vi "CommentSequenceFile.vi"(10 "Configuration File Path":path=path "CommentSequenceFile.Sample.ini", 11 "Sequence Context":refnum<k7>) -> ()   [LabVIEW 2017]
uses:
  <vilib>/Utility/config.llb/Read Key (String).vi
  <vilib>/Utility/config.llb/NI_LVConfig.lvlib
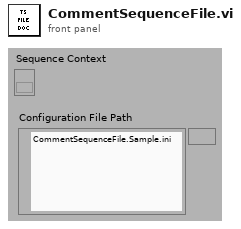
[diagram p1: front panel]
types:
  T1 = typedef "NI_LVConfig.lvlib/Config Data RefNum.ctl" = refnum<k1>
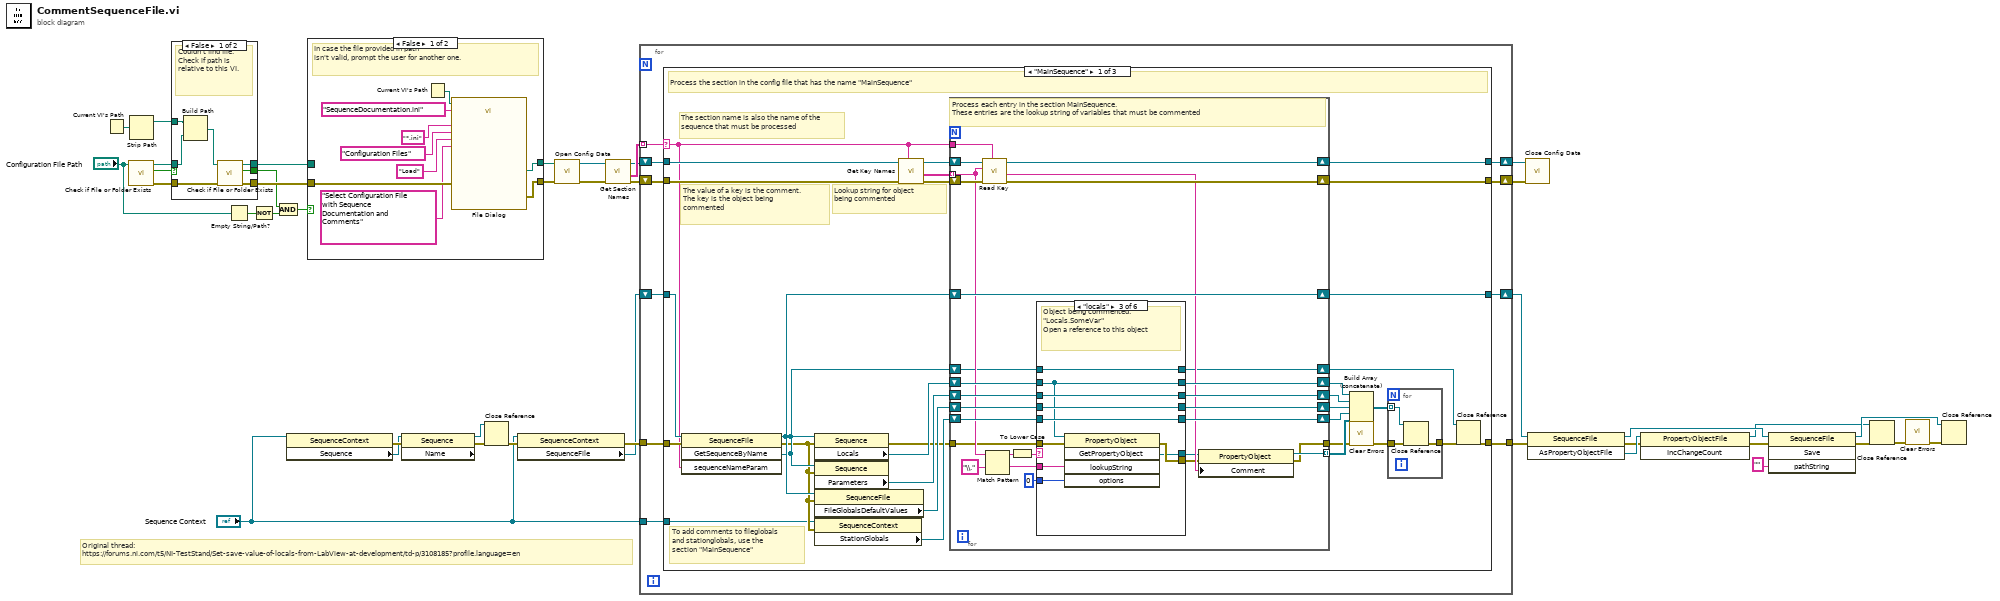
[diagram p0: block diagram]
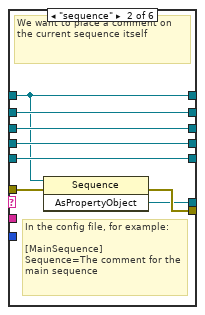
[diagram p4: hidden frame]
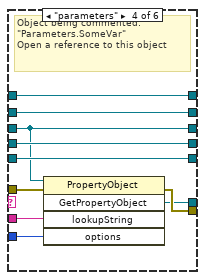
[diagram p5: hidden frame]
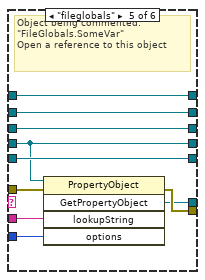
[diagram p6: hidden frame]
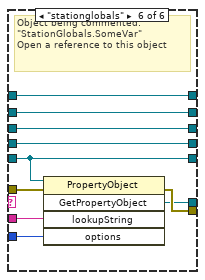
[diagram p7: hidden frame]
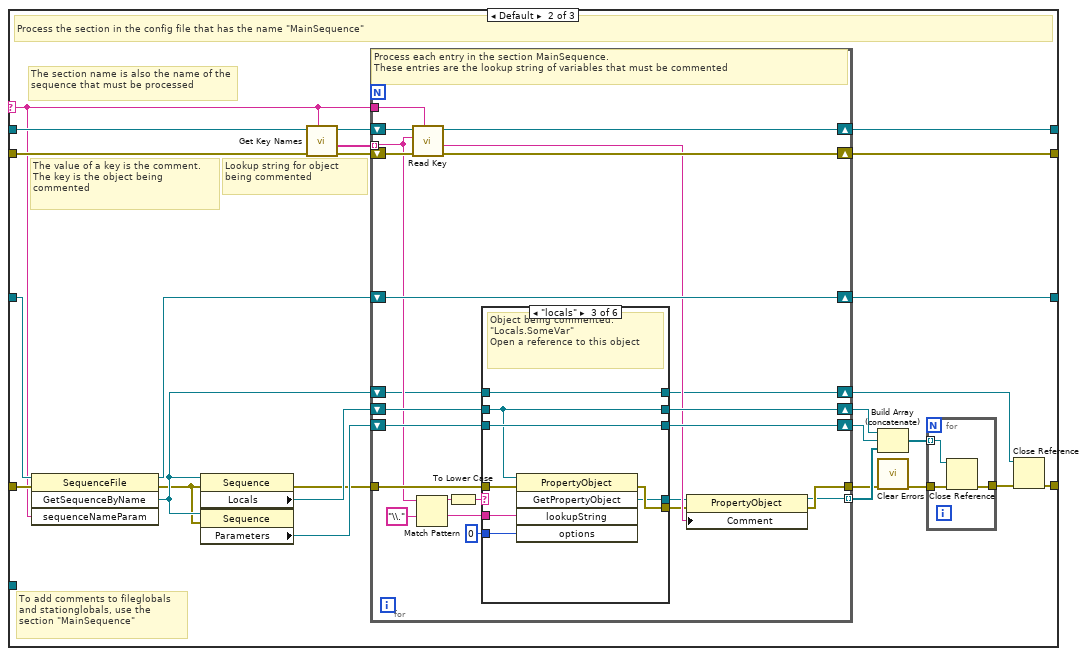
[diagram p8: hidden frame]
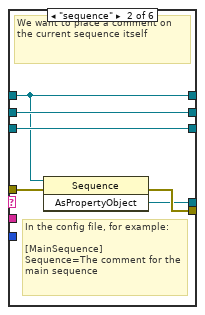
[diagram p10: hidden frame]
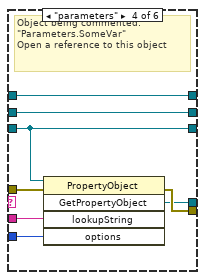
[diagram p11: hidden frame]
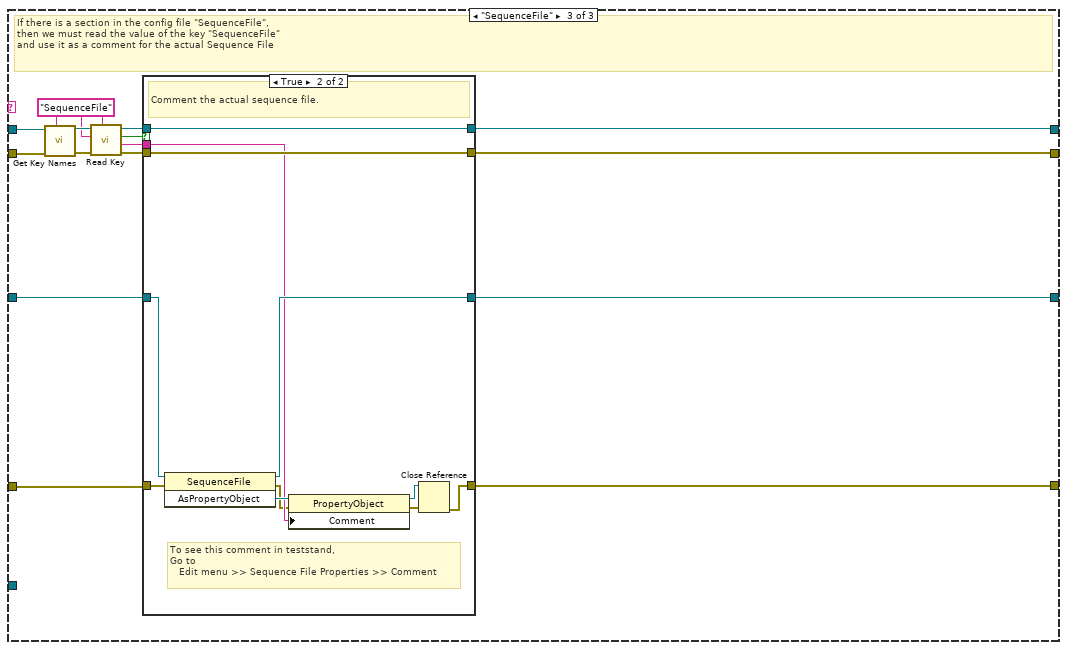
[diagram p14: hidden frame]
diagram:
  # "Original thread:\nhttps://forums.ni.com/t5/NI-TestStand/Set-save-value-of-locals-from-LabView-at-development/td-p/3108185?profile.language=en"
  n1 = Current VI's Path() -> (path=w2:path)
  n2 = call <vilib>:"Check if File or Folder Exists.vi"("path"="Configuration File Path") -> ("error out"=w7:errorcluster, "file or folder exists?"=w4:bool, "dup path"=w5:path)  [unwired: 8 in]
  n3 = Strip Path(path=w2) -> (stripped path=w1:path)  [unwired: 1 out]
  n4 = case shown="False" w4 {
    selector: w4 -> [_ w49]
    tunnel: [w46 w51] -> w8
    tunnel: w7 -> [w48 w51]
    tunnel: [w47 w50] -> w6
    tunnel: w5 -> [w43 w50]
    tunnel: [w45 w49] -> w3
    tunnel: w1 -> [w42 _]
    frame False {
      # "Couldn't find file.\nCheck if path is relative to this VI."
      n5 = Build Path(base path=w42, name or relative path=w43) -> (appended path=w44:path)
      n6 = call <vilib>:"Check if File or Folder Exists.vi"("error in (no error)"=w48, "path"=w44) -> ("error out"=w46:errorcluster, "file or folder exists?"=w45:bool, "dup path"=w47:path)  [unwired: 7 in]
    }
    frame True {
      # "Found file,\nNo worries"
    }
  }
  n7 = Empty String/Path?(string/path="Configuration File Path") -> (empty?=w12:bool)
  n8 = Not(x=w12) -> (.not. x?=w11:bool)
  n9 = And(x=w3, y=w11) -> (x .and. y?=w14:bool)
  n10 = property class="SequenceContext"(reference="Sequence Context") -> (error out=w30:errorcluster, "Sequence"=w24:refnum<k7>)  [unwired: 1 in, 1 out]
  n11 = case shown="False" w14 {
    tunnel: w6 -> [_ w62]
    tunnel: [w60 w62] -> w41
    tunnel: w8 -> [w58 w61]
    tunnel: [w59 w61] -> w40
    frame False {
      # "In case the file provided in path\nisn't valid, prompt the user for another one."
      n12 = Current VI's Path() -> (path=w57:path)
      n13 = call "File Dialog"("start path"=w57, "prompt"="Select Configuration File with Sequence Documentation and Comments", "button label"="Load", "default name"="SequenceDocumentation.ini", "error in"=w58, "pattern (all files)"="*.ini", "pattern label"="Configuration Files") -> ("selected path"=w60:path, "error out"=w59:errorcluster)  [unwired: 5 in, 2 out]
    }
    frame True {
      # "We have a valid file. No worries"
    }
  }
  n14 = property class="Sequence" props=["Name"](reference=w24, error in=w30) -> (reference out=w29:refnum<k7>, error out=w28:errorcluster)  [unwired: 1 out]
  n15 = Close Reference(reference=w29, error in (no error)=w28) -> (error out=w27:errorcluster)
  n16 = property class="SequenceContext"(reference="Sequence Context", error in=w27) -> (error out=w16:errorcluster, "SequenceFile"=w15:refnum<k7>)  [unwired: 1 out]
  n17 = call <vilib>:"Open Config Data.vi"("error in (no error)"=w40, "configuration file path"=w41) -> ("error out"=w21:errorcluster, "refnum"=w20:T1)  [unwired: 7 in, 1 out]
  n18 = call <vilib>:"Get Section Names.vi"("error in (no error)"=w21, "refnum"=w20) -> ("error out"=w17:errorcluster, "section names"=w19:string[], "refnum out"=w18:T1)  [unwired: 7 in]
  n19 = for {
    tunnel: "Sequence Context" -> [w68]
    shift-right: [w70] -> w25
    shift-left: w15 -> [w67]
    shift-right: [w72] -> w39
    shift-left: w17 -> [w65]
    shift-right: [w71] -> w38
    shift-left: w18 -> [w64]
    tunnel: w19 -> [w63] mode=indexing
    tunnel: w16 -> [w66]
    tunnel: [w69] -> w23
    n20 = case shown="\"MainSequence\"" w63 {
      selector: w63 -> [w79 w196 _]
      tunnel: [w102 w213 w278] -> w72
      tunnel: [w101 w212 w279] -> w71
      tunnel: [w98 w209 w277] -> w70
      tunnel: [w77 w193 w276] -> w69
      tunnel: w68 -> [w84 _ _]
      tunnel: w67 -> [w83 w200 w281]
      tunnel: w66 -> [w82 w199 w280]
      tunnel: w65 -> [w81 w198 w282]
      tunnel: w64 -> [w80 w197 w283]
      frame "MainSequence" {
        # "To add comments to fileglobals and stationglobals, use the section \"MainSequence\""
        # "Lookup string for object being commented"
        # "The value of a key is the comment. \nThe key is the object being commented"
        # "The section name is also the name of the sequence that must be processed"
        # "Process the section in the config file that has the name \"MainSequence\""
        n21 = invoke class="SequenceFile" method="GetSequenceByName"(reference=w83, error in=w82, "sequenceNameParam"=w79) -> (reference out=w96:refnum<k7>, error out=w85:errorcluster, "GetSequenceByName"=w86:refnum<k7>)  [unwired: 1 in, 1 out]
        n22 = property class="Sequence"(reference=w86, error in=w85) -> (error out=w75:errorcluster, "Locals"=w97:refnum<k7>)  [unwired: 1 out]
        n23 = property class="Sequence"(reference=w86, error in=w85) -> ("Parameters"=w95:refnum<k7>)  [unwired: 2 out]
        n24 = property class="SequenceFile"(reference=w96, error in=w85) -> ("FileGlobalsDefaultValues"=w94:refnum<k7>)  [unwired: 2 out]
        n25 = property class="SequenceContext"(reference=w84, error in=w85) -> ("StationGlobals"=w93:refnum<k7>)  [unwired: 2 out]
        n26 = call <vilib>:"Get Key Names.vi"("section"=w79, "error in (no error)"=w81, "refnum"=w80) -> ("error out"=w103:errorcluster, "key names"=w99:string[], "refnum out"=w100:T1)  [unwired: 5 in, 1 out]
        n27 = for {
          shift-right: [w131] -> w102
          shift-left: w103 -> [w134]
          shift-right: [w132] -> w101
          shift-left: w100 -> [w133]
          tunnel: w99 -> [w116] mode=indexing
          tunnel: w79 -> [w130]
          shift-right: [w127] -> w98
          shift-left: w96 -> [w127]
          shift-right: [w126] -> w92
          shift-left: w97 -> [w125]
          shift-right: [w120] -> w91
          shift-left: w93 -> [w119]
          shift-right: [w121] -> w90
          shift-left: w94 -> [w122]
          shift-right: [w124] -> w89
          shift-left: w95 -> [w123]
          tunnel: [w115] -> w88 mode=indexing
          shift-right: [w110] -> w76
          shift-left: w86 -> [w109]
          tunnel: w75 -> [w108]
          tunnel: [w107] -> w73
          # "Process each entry in the section MainSequence. \nThese entries are the lookup string of variables that must be commented"
          n28 = call-poly <vilib>:"Read Key.vi"("section"=w130, "error in (no error)"=w134, "key"=w116, "refnum"=w133) -> ("error out"=w131:errorcluster, "value"=w117:string, "refnum out"=w132:T1)  [unwired: 4 in, 1 out]
          n29 = Match Pattern(string=w116, regular expression="\\.") -> (before substring=w128:string, after substring=w114:string)  [unwired: 1 in, 2 out]
          n30 = To Lower Case(string=w128) -> (all lower case string=w118:string)
          n31 = case shown="\"locals\"" w118 {
            tunnel: [w136 w147 w150 w167 w177 w188] -> w126
            tunnel: w125 -> [w136 w147 w150 w167 w177 w188]
            tunnel: [w140 w146 w157 w165 w176 w186] -> w124
            tunnel: w123 -> [w140 w146 w157 w165 w176 w186]
            tunnel: w122 -> [w139 w142 w151 w166 w170 w187]
            tunnel: [w139 w142 w151 w166 w170 w187] -> w121
            tunnel: [w138 w148 w158 w168 w178 w180] -> w120
            tunnel: w119 -> [w138 w148 w158 w168 w178 w180]
            tunnel: [w137 w144 w155 w163 w174 w184] -> w111
            tunnel: w108 -> [w137 w145 w156 w164 w175 w185]
            tunnel: w114 -> [_ _ w154 w162 w173 w183]
            tunnel: 0 ("options") -> [_ _ w153 w161 w172 w182]
            tunnel: [_ w143 w152 w160 w171 w181] -> w112
            tunnel: [w135 w141 w149 w159 w169 w179] -> w110
            tunnel: w109 -> [w135 w141 w149 w159 w169 w179]
            frame Default {
              # "The object being commented does not belong to locals, fileglobals, stationglobals, or parameters.\n\nNote that form of the lookup string (from the keys in config file) must be of the form e.g.\n\nLocals.SomeVariable"
            }
            frame "sequence" {
              # "In the config file, for example:\n\n[MainSequence]\nSequence=The comment for the main sequence"
              # "We want to place a comment on the current sequence itself"
              n32 = invoke class="Sequence" method="AsPropertyObject"(reference=w141, error in=w145) -> (error out=w144:errorcluster, "AsPropertyObject"=w143:refnum<k7>)  [unwired: 1 in, 1 out]
            }
            frame "locals" {
              # "Object being commented:\n\"Locals.SomeVar\"\nOpen a reference to this object"
              n33 = invoke class="PropertyObject" method="GetPropertyObject"(reference=w150, error in=w156, "lookupString"=w154, "options"=w153) -> (error out=w155:errorcluster, "GetPropertyObject"=w152:refnum<k7>)  [unwired: 1 in, 3 out]
            }
            frame "parameters" {
              # "Object being commented:\n\"Parameters.SomeVar\"\nOpen a reference to this object"
              n34 = invoke class="PropertyObject" method="GetPropertyObject"(reference=w165, error in=w164, "lookupString"=w162, "options"=w161) -> (error out=w163:errorcluster, "GetPropertyObject"=w160:refnum<k7>)  [unwired: 1 in, 3 out]
            }
            frame "fileglobals" {
              # "Object being commented:\n\"FileGlobals.SomeVar\"\nOpen a reference to this object"
              n35 = invoke class="PropertyObject" method="GetPropertyObject"(reference=w170, error in=w175, "lookupString"=w173, "options"=w172) -> (error out=w174:errorcluster, "GetPropertyObject"=w171:refnum<k7>)  [unwired: 1 in, 3 out]
            }
            frame "stationglobals" {
              # "Object being commented:\n\"StationGlobals.SomeVar\"\nOpen a reference to this object"
              n36 = invoke class="PropertyObject" method="GetPropertyObject"(reference=w180, error in=w185, "lookupString"=w183, "options"=w182) -> (error out=w184:errorcluster, "GetPropertyObject"=w181:refnum<k7>)  [unwired: 1 in, 3 out]
            }
          }
          n37 = property class="PropertyObject"(reference=w112, error in=w111, "Comment"=w117) -> (reference out=w115:refnum<k7>, error out=w107:errorcluster)
        }
        n38 = Build Array (concatenate)(w92, w89, w90, w91, w88) -> (w87:refnum<k7>[])
        n39 = call <vilib>:"Clear Errors.vi"("error in (no error)"=w73) -> ("error out"=w74:errorcluster)  [unwired: 5 in, 1 out]
        n40 = for {
          tunnel: w87 -> [w106] mode=indexing
          tunnel: w74 -> [w105]
          tunnel: [w104] -> w78
          n41 = Close Reference(reference=w106, error in (no error)=w105) -> (error out=w104:errorcluster)
        }
        n42 = Close Reference(reference=w76, error in (no error)=w78) -> (error out=w77:errorcluster)
      }
      frame Default {
        # "To add comments to fileglobals and stationglobals, use the section \"MainSequence\""
        # "Lookup string for object being commented"
        # "The value of a key is the comment. \nThe key is the object being commented"
        # "The section name is also the name of the sequence that must be processed"
        # "Process the section in the config file that has the name \"MainSequence\""
        n43 = invoke class="SequenceFile" method="GetSequenceByName"(reference=w200, error in=w199, "sequenceNameParam"=w196) -> (reference out=w207:refnum<k7>, error out=w201:errorcluster, "GetSequenceByName"=w202:refnum<k7>)  [unwired: 1 in, 1 out]
        n44 = property class="Sequence"(reference=w202, error in=w201) -> (error out=w195:errorcluster, "Locals"=w208:refnum<k7>)  [unwired: 1 out]
        n45 = property class="Sequence"(reference=w202, error in=w201) -> ("Parameters"=w206:refnum<k7>)  [unwired: 2 out]
        n46 = call <vilib>:"Get Key Names.vi"("section"=w196, "error in (no error)"=w198, "refnum"=w197) -> ("error out"=w214:errorcluster, "key names"=w210:string[], "refnum out"=w211:T1)  [unwired: 5 in, 1 out]
        n47 = for {
          shift-right: [w238] -> w213
          shift-left: w214 -> [w241]
          shift-right: [w239] -> w212
          shift-left: w211 -> [w240]
          tunnel: w210 -> [w226] mode=indexing
          tunnel: w196 -> [w237]
          shift-right: [w234] -> w209
          shift-left: w207 -> [w234]
          shift-right: [w233] -> w205
          shift-left: w208 -> [w232]
          shift-right: [w231] -> w204
          shift-left: w206 -> [w230]
          tunnel: [w224] -> w191 mode=indexing
          shift-right: [w219] -> w192
          shift-left: w202 -> [w218]
          tunnel: w195 -> [w228]
          tunnel: [w225] -> w189
          # "Process each entry in the section MainSequence. \nThese entries are the lookup string of variables that must be commented"
          n48 = call-poly <vilib>:"Read Key.vi"("section"=w237, "error in (no error)"=w241, "key"=w226, "refnum"=w240) -> ("error out"=w238:errorcluster, "value"=w227:string, "refnum out"=w239:T1)  [unwired: 4 in, 1 out]
          n49 = Match Pattern(string=w226, regular expression="\\.") -> (before substring=w235:string, after substring=w223:string)  [unwired: 1 in, 2 out]
          n50 = To Lower Case(string=w235) -> (all lower case string=w229:string)
          n51 = case shown="\"locals\"" w229 {
            tunnel: [w243 w251 w253 w267 w271 w275] -> w233
            tunnel: w232 -> [w243 w251 w253 w267 w271 w275]
            tunnel: [w245 w250 w259 w266 w270 w274] -> w231
            tunnel: w230 -> [w245 w250 w259 w266 w270 w274]
            tunnel: [w244 w248 w257 w264 w269 w273] -> w220
            tunnel: w228 -> [w244 w249 w258 w265 w269 w273]
            tunnel: w223 -> [_ _ w256 w263 _ _]
            tunnel: 0 ("options") -> [_ _ w255 w262 _ _]
            tunnel: [_ w247 w254 w261 _ _] -> w221
            tunnel: [w242 w246 w252 w260 w268 w272] -> w219
            tunnel: w218 -> [w242 w246 w252 w260 w268 w272]
            frame Default {
              # "The object being commented does not belong to locals, fileglobals, stationglobals, or parameters.\n\nNote that form of the lookup string (from the keys in config file) must be of the form e.g.\n\nLocals.SomeVariable"
            }
            frame "sequence" {
              # "In the config file, for example:\n\n[MainSequence]\nSequence=The comment for the main sequence"
              # "We want to place a comment on the current sequence itself"
              n52 = invoke class="Sequence" method="AsPropertyObject"(reference=w246, error in=w249) -> (error out=w248:errorcluster, "AsPropertyObject"=w247:refnum<k7>)  [unwired: 1 in, 1 out]
            }
            frame "locals" {
              # "Object being commented:\n\"Locals.SomeVar\"\nOpen a reference to this object"
              n53 = invoke class="PropertyObject" method="GetPropertyObject"(reference=w253, error in=w258, "lookupString"=w256, "options"=w255) -> (error out=w257:errorcluster, "GetPropertyObject"=w254:refnum<k7>)  [unwired: 1 in, 3 out]
            }
            frame "parameters" {
              # "Object being commented:\n\"Parameters.SomeVar\"\nOpen a reference to this object"
              n54 = invoke class="PropertyObject" method="GetPropertyObject"(reference=w266, error in=w265, "lookupString"=w263, "options"=w262) -> (error out=w264:errorcluster, "GetPropertyObject"=w261:refnum<k7>)  [unwired: 1 in, 3 out]
            }
            frame "fileglobals" {
              # "We will only comment station globals from the \"MainSequence\" section in the config file"
            }
            frame "stationglobals" {
              # "We will only comment station globals from the \"MainSequence\" section in the config file"
            }
          }
          n55 = property class="PropertyObject"(reference=w221, error in=w220, "Comment"=w227) -> (reference out=w224:refnum<k7>, error out=w225:errorcluster)
        }
        n56 = Build Array (concatenate)(w205, w204, w191) -> (w203:refnum<k7>[])
        n57 = call <vilib>:"Clear Errors.vi"("error in (no error)"=w189) -> ("error out"=w190:errorcluster)  [unwired: 5 in, 1 out]
        n58 = for {
          tunnel: w203 -> [w217] mode=indexing
          tunnel: w190 -> [w216]
          tunnel: [w215] -> w194
          n59 = Close Reference(reference=w217, error in (no error)=w216) -> (error out=w215:errorcluster)
        }
        n60 = Close Reference(reference=w192, error in (no error)=w194) -> (error out=w193:errorcluster)
      }
      frame "SequenceFile" {
        w288 = "SequenceFile" ("section")
        # "If there is a section in the config file \"SequenceFile\", \nthen we must read the value of the key \"SequenceFile\" \nand use it as a comment for the actual Sequence File"
        n61 = call <vilib>:"Get Key Names.vi"("section"=w288, "error in (no error)"=w282, "refnum"=w283) -> ("error out"=w290:errorcluster, "refnum out"=w289:T1)  [unwired: 5 in, 2 out]
        n62 = call-poly <vilib>:"Read Key.vi"("section"=w288, "error in (no error)"=w290, "key"=w288, "refnum"=w289) -> ("error out"=w285:errorcluster, "value"=w284:string, "found?"=w287:bool, "refnum out"=w286:T1)  [unwired: 4 in]
        n63 = case shown="True" w287 {
          tunnel: [w293 w305] -> w279
          tunnel: w286 -> [w293 w305]
          tunnel: [w294 w304] -> w278
          tunnel: w285 -> [w294 w304]
          tunnel: w281 -> [w292 w303]
          tunnel: w280 -> [w291 w302]
          tunnel: [w292 w301] -> w277
          tunnel: w284 -> [_ w299]
          tunnel: [w291 w295] -> w276
          frame False {
            # "There is no comment for the actual sequence file"
          }
          frame True {
            # "To see this comment in teststand, \nGo to \n   Edit menu >> Sequence File Properties >> Comment"
            # "Comment the actual sequence file."
            n64 = invoke class="SequenceFile" method="AsPropertyObject"(reference=w303, error in=w302) -> (reference out=w301:refnum<k7>, error out=w297:errorcluster, "AsPropertyObject"=w300:refnum<k7>)  [unwired: 1 in]
            n65 = property class="PropertyObject"(reference=w300, error in=w297, "Comment"=w299) -> (reference out=w296:refnum<k7>, error out=w298:errorcluster)
            n66 = Close Reference(reference=w296, error in (no error)=w298) -> (error out=w295:errorcluster)
          }
        }
      }
    }
  }
  n67 = call <vilib>:"Close Config Data.vi"("error in (no error)"=w39, "refnum"=w38) -> ()  [unwired: 8 in, 2 out]
  n68 = invoke class="SequenceFile" method="AsPropertyObjectFile"(reference=w25, error in=w23) -> (reference out=w36:refnum<k7>, error out=w31:errorcluster, "AsPropertyObjectFile"=w37:refnum<k7>)  [unwired: 1 in]
  n69 = invoke class="PropertyObjectFile" method="IncChangeCount"(reference=w37, error in=w31) -> (reference out=w32:refnum<k7>, error out=w34:errorcluster)  [unwired: 1 in, 1 out]
  n70 = invoke class="SequenceFile" method="Save"(reference=w36, error in=w34, "pathString"="") -> (reference out=w33:refnum<k7>, error out=w26:errorcluster)  [unwired: 1 in, 2 out]
  n71 = Close Reference(reference=w32, error in (no error)=w26) -> (error out=w10:errorcluster)
  n72 = call <vilib>:"Clear Errors.vi"("error in (no error)"=w10) -> ("error out"=w9:errorcluster)  [unwired: 5 in, 1 out]
  n73 = Close Reference(reference=w33, error in (no error)=w9) -> ()  [unwired: 1 out]
